vi "Global_Hopper Statis.vi"() -> ()   [LabVIEW 2017, in "Hopper System.lvlib"]
uses:
  Systems/Hopper/Hopper System.lvlib
  Systems/Hopper/ENUM_State.ctl
  Systems/Hopper/ENUM_Action.ctl
panel:
  out "Hopper Complete_SM":bool
  in  "Hopper Action":T1
  in  "Hopper State":T2
  out "Hopper Empty Hopper_HW":bool
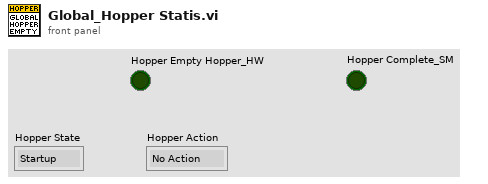
[diagram p1: front panel]
types:
  T1 = typedef "Hopper System.lvlib/ENUM_Action.ctl" = enum16{"No Action", "Reset Time", "Check Time Loading", "Check Time Rapid", "Reset All", "Loader Run", "Reset Loader", "Reset Counter", "Check Counter", "Inner Motor Run", "Reset Inner Motor", "Reset Shooting", "Shooting Complete"}
  T2 = typedef "Hopper System.lvlib/ENUM_State.ctl" = enum16{"Startup", "Idle", "Loading", "Ball Ready", "Shotgun Fire", "Rapid Fire", "5 Second", "Hopper E-STOP", "Shutdown"}
diagram:
